vi "Sig2MS catptureInformation.vi"(8 "error in (no error)":errorcluster, 9 "Index":i32, 11 "Sig2MS in":refnum<class "Sig2MS.lvclass">) -> (0 "error out":errorcluster, 1 "SectionalSig":waveform(sgl), 3 "Sig2MS out":refnum<class "Sig2MS.lvclass">, 5 "Label":string)   [LabVIEW 2018, in "Sig2MS.lvclass"]
uses:
  Sig2MS.lvclass
  Sig2MS.lvclass/Sig2MS.ctl
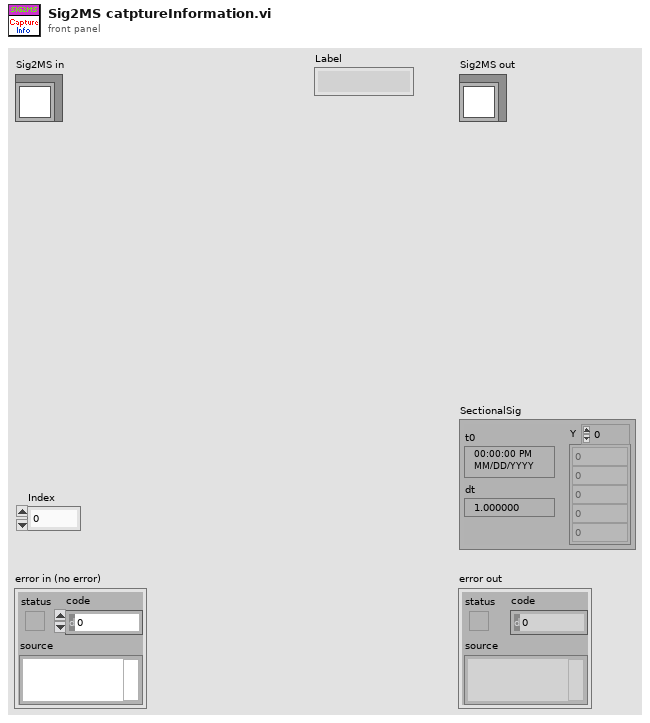
[diagram p1: front panel]
types:
  T1 = cluster{"Label":string, "dt":dbl, "Length":u32, "RefVolt":dbl, "mzTable":cluster{"t":dbl[], "mz":dbl[], "beta":dbl[]}}[]
  T2 = cluster{"Label":string, "dt":dbl, "Length":u32, "RefVolt":dbl, "mzTable":cluster{"t":dbl[], "mz":dbl[], "beta":dbl[]}}
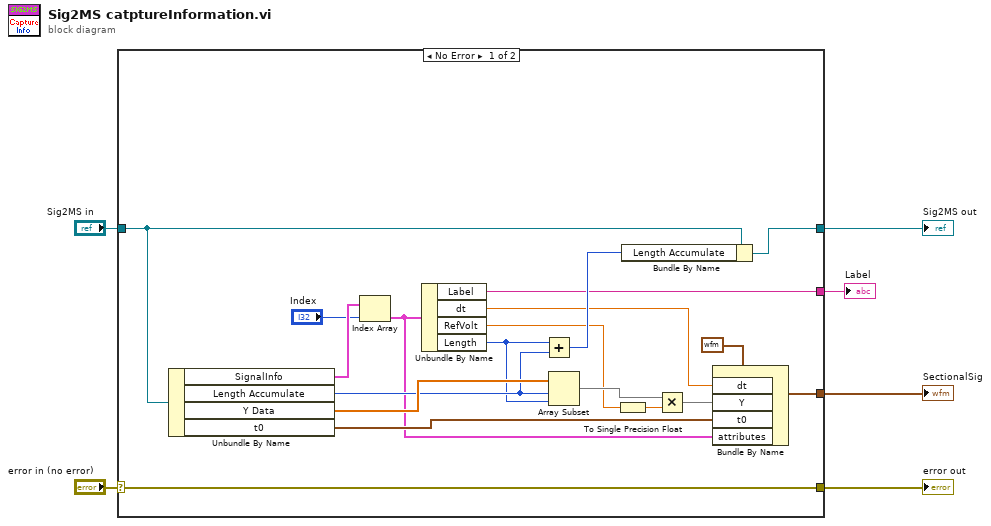
[diagram p0: block diagram]
diagram:
  n1 = case shown="No Error" "error in (no error)" {
    selector: "error in (no error)" -> [w25 w27]
    tunnel: [w25 w27] -> w5
    tunnel: [w16 w26] -> w3
    tunnel: "Sig2MS in" -> [w8 w26]
    tunnel: [w17 _] -> w1
    tunnel: [w9 _] -> w2
    frame No Error {
      n2 = Unbundle By Name(w8) -> ("SignalInfo"=w24:T1, "Length Accumulate"=w22:u32, "Y Data"=w23:sgl[], "t0"=w18:timestamp)
      n3 = Index Array(array=w24, index="Index") -> (element=w10:T2)
      n4 = Unbundle By Name(w10) -> ("Label"=w9:string, "dt"=w7:dbl, "RefVolt"=w12:dbl, "Length"=w13:u32)
      n5 = Add(x=w13, y=w22) -> (x+y=w15:u32)
      n6 = Array Subset(array=w23, index=w22, length=w13) -> (w21:sgl[])
      n7 = To Single Precision Float(number=w12) -> (single precision float=w11:sgl)
      n8 = Bundle By Name(cluster=w8, "Length Accumulate"=w15) -> (w16:refnum<class "Sig2MS.lvclass">)
      n9 = Multiply(x=w21, y=w11) -> (x*y=w19:sgl[])
      n10 = Bundle By Name(cluster=waveform(sgl) {"t0"=timestamp(0 s since 1904-01-01), "dt"=1.0, "Y"=[]} ("output waveform"), "dt"=w7, "Y"=w19, "t0"=w18, "attributes"=w10) -> (w17:waveform(sgl))
    }
    frame Error {
    }
  }
  "error out" <- w5
  "Sig2MS out" <- w3
  "SectionalSig" <- w1
  "Label" <- w2
